vi "TestConfig.vi"(8 "error in":errorcluster {"code" format="Error %.0f"}, 11 "MainFGV_data":T2={"TestDir"=path "", "TestName"="", "task"="", "data_file"=refnum, "burts_file"=refnum, "log_file"=refnum, "AcqQueue"=refnum, "StartTime"=timestamp(0 s since 1904-01-01), "config_channels"=[], "DAQmx Device"="", "Advanced"={"rate"=1652.0, "duration"=1.0, "thr"=100.0, "preTrigger"=100.0, "cutoff"=-3.0, "Filtro"=enum."Desativado", "highPass"=1000.0, "lowPass"=1000.0, "updateTime"=50.0}, "running"=FALSE} {"Advanced"."updateTime" format="%#_g ms"; "Advanced"."lowPass" format="%#_g Hz"; "Advanced"."highPass" format="%#_g Hz"; "Advanced"."cutoff" format="%#_g dB"; "Advanced"."preTrigger" format="%#_g ms"; "Advanced"."thr" format="%#_g N"; "Advanced"."duration" format="%#_g s"; "Advanced"."rate" min=1652.0 max=51200.0 format="%#_g Hz"}) -> (0 "error out":errorcluster {"code" format="Error %.0f"}, 3 "MainFGV_data out":T2={"TestDir"=path "", "TestName"="", "task"="", "data_file"=refnum, "burts_file"=refnum, "log_file"=refnum, "AcqQueue"=refnum, "StartTime"=timestamp(0 s since 1904-01-01), "config_channels"=[], "DAQmx Device"="", "Advanced"={"rate"=1652.0, "duration"=1.0, "thr"=100.0, "preTrigger"=100.0, "cutoff"=-3.0, "Filtro"=enum."Desativado", "highPass"=1000.0, "lowPass"=1000.0, "updateTime"=50.0}, "running"=FALSE} {"Advanced"."updateTime" format="%#_g ms"; "Advanced"."lowPass" format="%#_g Hz"; "Advanced"."highPass" format="%#_g Hz"; "Advanced"."cutoff" format="%#_g dB"; "Advanced"."preTrigger" format="%#_g ms"; "Advanced"."thr" format="%#_g N"; "Advanced"."duration" format="%#_g s"; "Advanced"."rate" min=1652.0 max=51200.0 format="%#_g Hz"})   [LabVIEW 2016]
uses:
  MainFGV_data.ctl
  config_board.ctl
  Advanced/AdvancedConfig.ctl
  Log/log_mods.ctl
  Log/log_status.ctl
panel:
  in  "config":T1[](array[typedef]) caption="Configurações"
  in  "DAQmx Device":tag
  in  "OK":bool
  in  "Cancelar":bool
  in  "OpenConfig":bool caption="Abrir\nconfiguração"
  in  "SaveConfig":bool caption="Salvar\nconfiguração"
  # "Configuração dos canais para o ensaio"
  # "Sensibilidade:\nMartelo - mV/N\nAcelerômetro - mV/g"
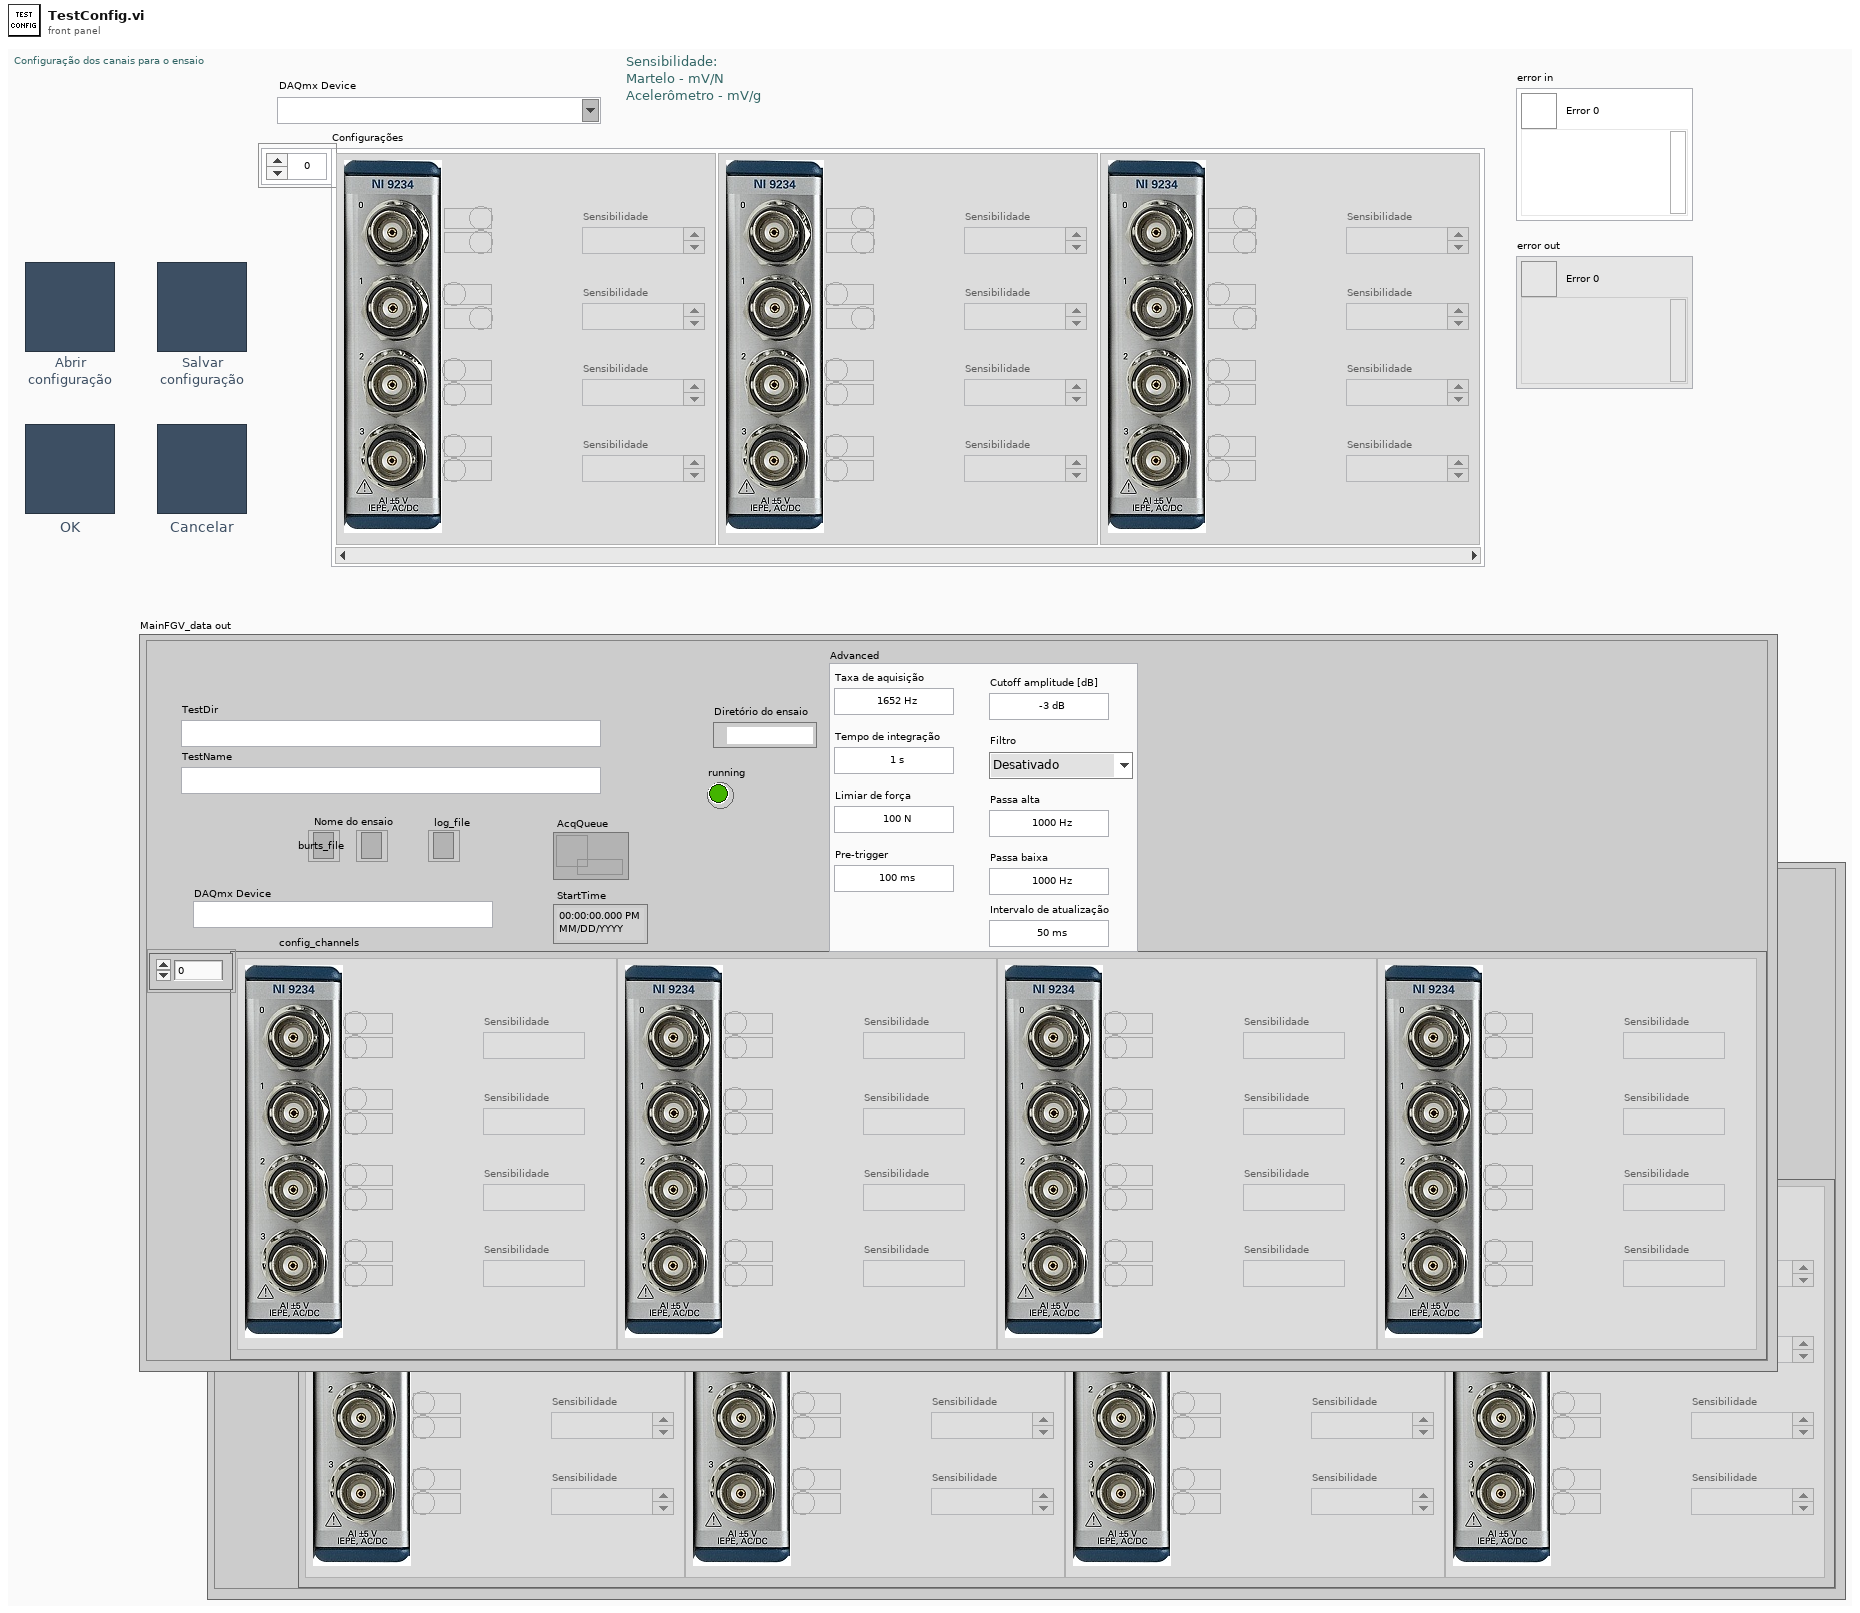
[diagram p1: front panel]
types:
  T1 = typedef "config_board.ctl" = cluster{"Sens 1":dbl, "active 1":bool, "type 1":bool, "type 2":bool, "active 2":bool, "Sens 2":dbl, "type 3":bool, "active 3":bool, "Sens 3":dbl, "type 4":bool, "active 4":bool, "Sens 4":dbl}
  T2 = typedef "MainFGV_data.ctl" = cluster{"TestDir":path, "TestName":string, "task":refnum<k21>, "data_file":refnum<file>, "burts_file":refnum<file>, "log_file":refnum<file>, "AcqQueue":refnum<queue>, "StartTime":timestamp, "config_channels":T1[], "DAQmx Device":tag, "Advanced":T3, "running":bool}
  T3 = typedef "AdvancedConfig.ctl" = cluster{"rate":dbl, "duration":dbl, "thr":dbl, "preTrigger":dbl, "cutoff":dbl, "Filtro":enum16{"Desativado", "Passa banda", "Passa alta", "Passa baixa"}, "highPass":dbl, "lowPass":dbl, "updateTime":dbl}
  T4 = typedef "log_status.ctl" = enum16{"Init", "Ready", "Running", "Error", "End"}
  T5 = typedef "log_mods.ctl" = enum16{"Init", "LogFileRefnum", "SetStatus", "WriteAcel", "WriteToLog", "End"}
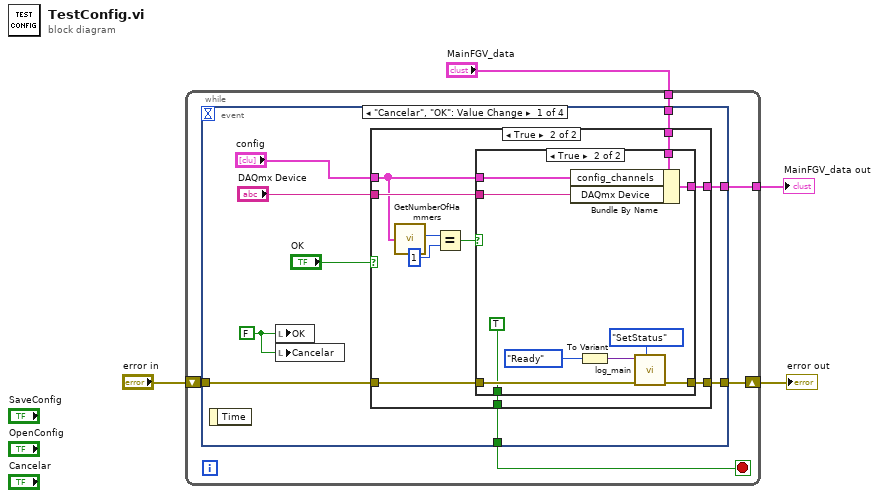
[diagram p0: block diagram]
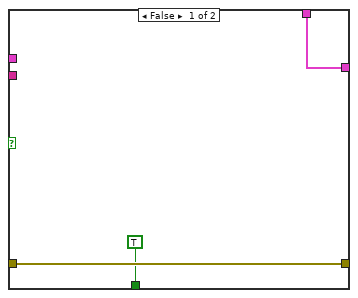
[diagram p2: hidden frame]
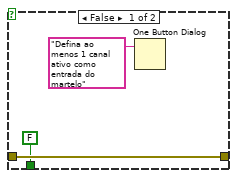
[diagram p3: hidden frame]
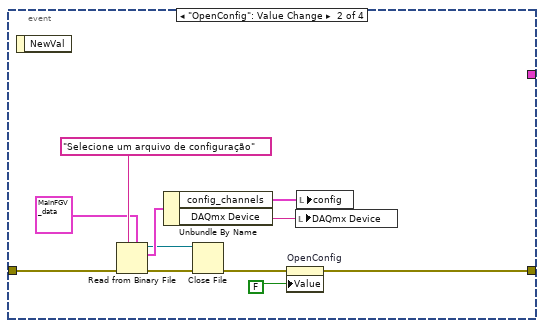
[diagram p4: hidden frame]
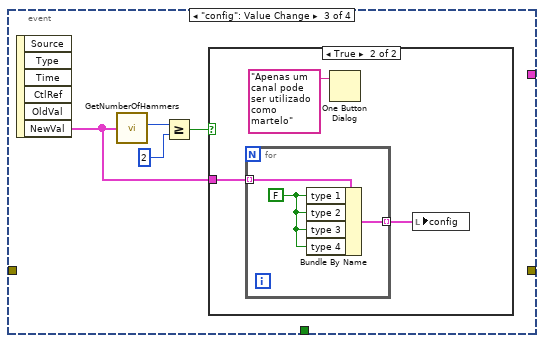
[diagram p5: hidden frame]
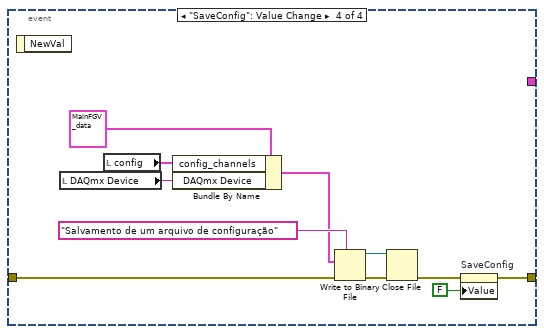
[diagram p7: hidden frame]
diagram:
  n1 = while {
    shift-right: [w7] -> w3
    shift-left: "error in" -> [w8]
    tunnel: "MainFGV_data" -> [w6]
    tunnel: [w5] -> w1
    stop <- w9 stop-if-true
    n2 = event shown="[0] \"Cancelar\", \"OK\": Value Change" {
      selector: _ -> [_ _ _ _]
      dyn-events: _ -> [_ _ _ _]
      timeout: _ -> [_ _ _ _]
      tunnel: [w10 _ _ _] -> w9
      tunnel: w8 -> [w14 w54 _ w72]
      tunnel: [w13 w45 _ w67] -> w7
      tunnel: w6 -> [w18 _ _ _]
      tunnel: [w17 _ _ _] -> w5
      event "Cancelar", "OK": Value Change {
        w16 = FALSE ("OK")
        n3 = event-data() -> ()  [unwired: 1 in, 1 out]
        n4 = local write "OK"(w16) -> ()
        n5 = local write "Cancelar"(w16) -> ()
        n6 = case shown="True" "OK" {
          tunnel: "DAQmx Device" -> [_ w31]
          tunnel: "config" -> [_ w26]
          tunnel: w18 -> [w21 w30]
          tunnel: [w21 w29] -> w17
          tunnel: w14 -> [w20 w28]
          tunnel: [w20 w27] -> w13
          tunnel: [TRUE ("OK") w22] -> w10
          frame False {
          }
          frame True {
            n7 = call "GetNumberOfHammers.vi"("config"=w26) -> ("hammers"=w25:i16)  [unwired: 8 in, 1 out]
            n8 = Equal?(x=w25, y=i16 1) -> (x = y?=w24:bool)
            n9 = case shown="True" w24 {
              tunnel: w31 -> [_ w44]
              tunnel: w26 -> [_ w43]
              tunnel: w30 -> [_ w42]
              tunnel: [_ w41] -> w29
              tunnel: w28 -> [w33 w37]
              tunnel: [w33 w36] -> w27
              tunnel: [FALSE ("OK") TRUE ("OK")] -> w22
              frame False {
                n10 = One Button Dialog(message="Defina ao menos 1 canal ativo como entrada do martelo") -> ()  [unwired: 1 in, 1 out]
              }
              frame True {
                n11 = Bundle By Name(cluster=w42, "config_channels"=w43, "DAQmx Device"=w44) -> (w41:T2)
                n12 = To Variant(anything=log_status."Ready" ("log_status")) -> (Variant=w38:variant)
                n13 = call "log_main.vi"("FGV_mods"=log_mods."SetStatus", "Error In"=w37, "DataIn"=w38) -> ("Error Out"=w36:errorcluster)  [unwired: 7 in, 1 out]
              }
            }
          }
        }
      }
      event "OpenConfig": Value Change {
        n14 = event-data() -> ()  [unwired: 1 in, 1 out]
        n15 = Read from Binary File(5:T2 {"TestDir"=path "C:/Users/l01481/Desktop/Teste_0", "TestName"="Teste", "task"="", "data_file"=refnum, "burts_file"=refnum, "log_file"=refnum, "AcqQueue"=refnum, "StartTime"=timestamp(0 s since 1904-01-01), "config_channels"=[], "DAQmx Device"="", "Advanced"={"rate"=1652.0, "duration"=1.0, "thr"=100.0, "preTrigger"=100.0, "cutoff"=-3.0, "Filtro"=enum."Desativado", "highPass"=1000.0, "lowPass"=1000.0, "updateTime"=50.0}, "running"=FALSE} ("MainFGV_data"), 7:"Selecione um arquivo de configuração" ("prompt (Open existing file)"), 8:w54) -> (0:w51:errorcluster, 2:w52:T2, 3:w50:refnum<file>)  [unwired: 3 in, 1 out]
        n16 = Unbundle By Name(w52) -> ("config_channels"=w48:T1[], "DAQmx Device"=w49:tag)
        n17 = Close File(refnum=w50, error in=w51) -> (error out=w46:errorcluster)  [unwired: 1 out]
        n18 = property on="OpenConfig" class="Bool (strict)"(error in=w46, "Value"=FALSE ("SaveConfig")) -> (error out=w45:errorcluster)  [unwired: 1 in, 1 out]
        n19 = local write "DAQmx Device"(w49) -> ()
        n20 = local write "config"(w48) -> ()
      }
      event "config": Value Change {
        n21 = event-data() -> ("NewVal"=w56:T1[])  [unwired: 1 in, 5 out]
        n22 = call "GetNumberOfHammers.vi"("config"=w56) -> ("hammers"=w59:i16)  [unwired: 8 in, 1 out]
        n23 = Greater Or Equal?(x=w59, y=i16 2) -> (x >= y?=w57:bool)
        n24 = case shown="True" w57 {
          tunnel: w56 -> [_ w61]
          frame False {
          }
          frame True {
            n25 = for {
              tunnel: w61 -> [w65] mode=indexing
              tunnel: [w63] -> w60 mode=indexing
              w64 = FALSE ("type 1")
              n26 = Bundle By Name(cluster=w65, "type 1"=w64, "type 2"=w64, "type 3"=w64, "type 4"=w64) -> (w63:T1)
            }
            n27 = One Button Dialog(message="Apenas um canal pode ser utilizado como martelo") -> ()  [unwired: 1 in, 1 out]
            n28 = local write "config"(w60) -> ()
          }
        }
      }
      event "SaveConfig": Value Change {
        n29 = event-data() -> ()  [unwired: 1 in, 1 out]
        n30 = local read "DAQmx Device"() -> (w74:tag)
        n31 = local read "config"() -> (w75:T1[])
        n32 = Bundle By Name(cluster=T2 {"TestDir"=path "C:/Users/l01481/Desktop/Teste_0", "TestName"="Teste", "task"="", "data_file"=refnum, "burts_file"=refnum, "log_file"=refnum, "AcqQueue"=refnum, "StartTime"=timestamp(0 s since 1904-01-01), "config_channels"=[], "DAQmx Device"="", "Advanced"={"rate"=1652.0, "duration"=1.0, "thr"=100.0, "preTrigger"=100.0, "cutoff"=-3.0, "Filtro"=enum."Desativado", "highPass"=1000.0, "lowPass"=1000.0, "updateTime"=50.0}, "running"=FALSE} ("MainFGV_data"), "config_channels"=w75, "DAQmx Device"=w74) -> (w69:T2)
        n33 = Write to Binary File(data=w69, error in=w72, 7:"Salvamento de um arquivo de configuração" ("prompt (Choose or enter file path)")) -> (refnum out=w70:refnum<file>, error out=w71:errorcluster)  [unwired: 3 in, 1 out]
        n34 = Close File(refnum=w70, error in=w71) -> (error out=w68:errorcluster)  [unwired: 1 out]
        n35 = property on="SaveConfig" class="Bool (strict)"(error in=w68, "Value"=FALSE ("SaveConfig")) -> (error out=w67:errorcluster)  [unwired: 1 in, 1 out]
      }
    }
  }
  "MainFGV_data out" <- w1
  "error out" <- w3
